vi "Get Result.vi"(8 "error in (no error)":errorcluster, 11 "LR-700 in":refnum<class "LR-700 Driver.lvclass">=refnum) -> (0 "error out":errorcluster, 2 "Result":refnum<class "Acquired Result.lvclass">, 3 "LR-700 out":refnum<class "LR-700 Driver.lvclass">)   [LabVIEW 2016, in "LR-700 Driver.lvclass"]
uses:
  LR-700 Driver.lvclass
  C:/github/NHMFL_Core/Libraries/Instruments/VISA Instrument/VISA Instrument.lvclass
  C:/github/NHMFL_Core/Libraries/Instruments/Instrument Driver/Channel Scanner Driver/Channel Scanner Driver.lvclass
  C:/github/NHMFL_Core/Libraries/Instruments/Instrument Driver/Instrument Driver.lvclass
  Measure_core/Results/Acquired Result/Acquired Result.lvclass
  Measure_core/Results/Acquired Result/Acquired Result.lvclass/Acquired Result.ctl
  VISA Instrument/VISA Instrument.lvclass/VISA Instrument.ctl
  Instrument Driver/Channel Scanner Driver/Channel Scanner Driver.lvclass/Channel Scanner Driver.ctl
  Instrument Driver/Instrument Driver.lvclass/Instrument Driver.ctl
  Measure_core/Results/Acquired Result/Read Group.vi
  VISA Instrument/Read VISA resource.vi
  Instrument Driver/Channel Scanner Driver/Read Scan Channels.vi
  Instrument Driver/Read Recorder name.vi
  VISA Instrument/Write VISA resource.vi
  Measure_core/Results/Acquired Result/Write Group.vi
  <vilib>/express/express shared/transition.llb/Dynamic To Waveform Array.vi
  <vilib>/express/express signal manip/GetorSetDDTAttributes/Set DDT Attributes/SetT0.vi
  <vilib>/express/express shared/transition.llb/Waveform Array To Dynamic.vi
  <vilib>/express/express signal manip/GetorSetDDTAttributes/Set DDT Attributes/Set DDT Properties.xnode
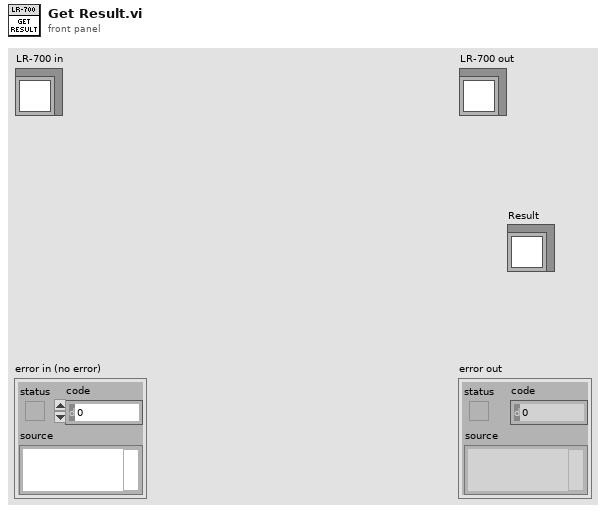
[diagram p1: front panel]
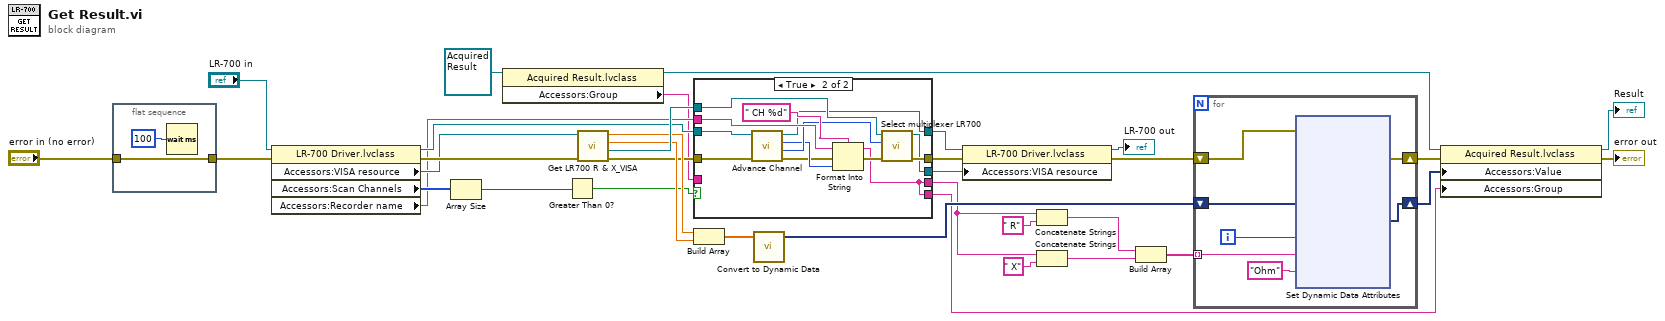
[diagram p0: block diagram]
diagram:
  n1 = flat-sequence {
    tunnel: "error in (no error)" -> [w37]
    tunnel: [w37] -> w24
    frame #0 {
      n2 = Wait (ms)(milliseconds to wait=u32 100) -> ()  [unwired: 1 out]
    }
  }
  n3 = property class="LR-700 Driver.lvclass"(reference="LR-700 in", error in=w24) -> (reference out=w22:refnum<class "LR-700 Driver.lvclass">, error out=w35:errorcluster, "Accessors:VISA resource"=w23:refnum<visa-resource-name>, "Accessors:Scan Channels"=w19:i32[], "Accessors:Recorder name"=w18:string)
  n4 = Array Size(array=w19) -> (size(s)=w30:i32)
  n5 = property class="Acquired Result.lvclass"(reference=refnum<class "Acquired Result.lvclass"> refnum ("Result")) -> (reference out=w1:refnum<class "Acquired Result.lvclass">, "Accessors:Group"=w2:string)  [unwired: 1 in, 1 out]
  n6 = Greater Than 0?(x=w30) -> (x > 0?=w27:bool)
  n7 = call "Get LR700 R & X_VISA.vi"("error in (no error)"=w35, "VISA resource name"=w23) -> ("error out"=w29:errorcluster, "VISA resource name out"=w33:refnum<visa-resource-name>, "X"=w31:dbl, "Resistance"=w32:dbl)  [unwired: 2 in]
  n8 = case shown="True" w27 {
    tunnel: w33 -> [w42 w51]
    tunnel: [w42 w50] -> w20
    tunnel: w22 -> [w39 w48]
    tunnel: w18 -> [w41 w55]
    tunnel: [w41 w49] -> w5
    tunnel: w29 -> [w40 w44]
    tunnel: [w40 w52] -> w28
    tunnel: [w39 w47] -> w21
    tunnel: [w38 w49] -> w4
    tunnel: w2 -> [w38 _]
    frame False {
    }
    frame True {
      n9 = call-dynamic "Advance Channel.vi"("error in (no error)"=w44, "Channel Scanner Driver in"=w48) -> ("error out"=w43:errorcluster, "Next channel"=w46:i32, "Current channel"=w45:i32, "Channel Scanner Driver out"=w47:refnum<class "LR-700 Driver.lvclass">)  [unwired: 6 in]
      n10 = Format Into String(format string=" CH %d", initial string=w55, error in=w43, w45) -> (resulting string=w49:string, error out=w53:errorcluster)
      n11 = call "Select multiplexer LR700.vi"("error in"=w53, "Sensor <01-99>"=w46, "VISA Resource Name"=w51) -> ("error out"=w52:errorcluster, "VISA Resource Name Out"=w50:refnum<visa-resource-name>)  [unwired: 7 in]
    }
  }
  n12 = Build Array(w32, w31) -> (w17:dbl[])
  n13 = call "Convert to Dynamic Data"("Array"=w17) -> ("Dynamic Data Type"=w12:dynamicdata)  [unwired: 3 in]
  n14 = property class="LR-700 Driver.lvclass"(reference=w21, error in=w28, "Accessors:VISA resource"=w20) -> (reference out=→"LR-700 out":refnum<class "LR-700 Driver.lvclass">, error out=w10:errorcluster)
  n15 = Concatenate Strings(w5, " R") -> (w14:string)
  n16 = Concatenate Strings(w5, " X") -> (w13:string)
  n17 = Build Array(w14, w13) -> (w11:string[])
  n18 = for {
    shift-right: [w59] -> w6
    shift-left: w12 -> [w60]
    tunnel: w11 -> [w58] mode=indexing
    shift-right: [w61] -> w9
    shift-left: w10 -> [w62]
    i -> [w56]
    n19 = xnode "Set Dynamic Data Attributes"("Signals In"=w60, "Signal Index"=w56, "Signal Name"=w58, "Unit"="Ohm", "error in"=w62) -> ("Signals Out"=w59:dynamicdata, "error out"=w61:errorcluster)
  }
  n20 = property class="Acquired Result.lvclass"(reference=w1, error in=w9, "Accessors:Value"=w6, "Accessors:Group"=w4) -> (reference out=→"Result":refnum<class "Acquired Result.lvclass">, error out=→"error out":errorcluster)
